vi "Main.vi"() -> ()   [LabVIEW 2013]
uses:
  ApplicationInititialisationClass/ApplicationInititialisation.lvclass
panel:
  out "error out":errorcluster
  out "Ergebnis-String":string
  out "VI-Name":string
  out "VI-Pfad":path
  out "WhereIGetMyInformation":string
  out "WhoIAm":string
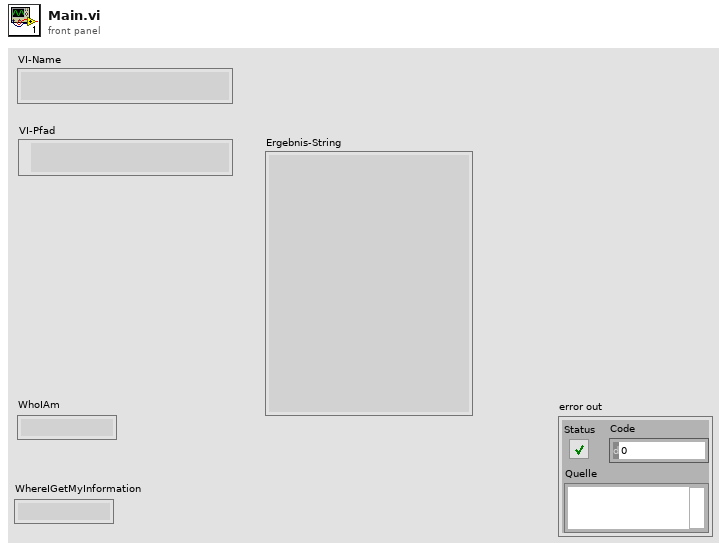
[diagram p1: front panel]
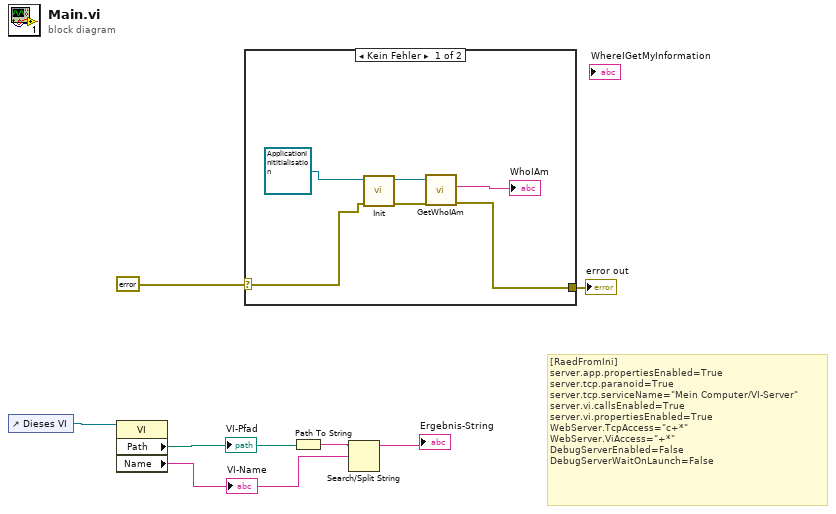
[diagram p0: block diagram]
diagram:
  # "[RaedFromIni]\nserver.app.propertiesEnabled=True\nserver.tcp.paranoid=True\nserver.tcp.serviceName=\"Mein Computer/VI-Server\"\nserver.vi.callsEnabled=True\nserver.vi.propertiesEnabled=True\nWebServer.TcpAccess=\"c+*\"\nWebServer.ViAccess=\"+*\"\nDebugServerEnabled=False\nDebugServerWaitOnLaunch=False"
  n1 = control-ref of="Dieses VI"() -> (w7:refnum<vi>)
  n2 = property class="VI"(reference=w7) -> ("Path"=w6:path, "Name"=w4:string)  [unwired: 1 in, 2 out]
  "VI-Pfad" <- w6
  "VI-Name" <- w4
  n3 = case shown="Kein Fehler" errorcluster {"status"=FALSE, "code"=0, "source"=""} ("error in (no error)") {
    selector: errorcluster {"status"=FALSE, "code"=0, "source"=""} ("error in (no error)") -> [w8 w14]
    tunnel: [w12 w14] -> w1
    frame No Error {
      n4 = call-dynamic "Init.vi"("error in (no error)"=w8, "ApplicationInititialisation Eingang"=refnum<class "ApplicationInititialisation.lvclass"> refnum ("ApplicationInititialisation.lvclass")) -> ("error out"=w9:errorcluster, "ApplicationInititialisation Ausgang"=w10:refnum<class "ApplicationInititialisation.lvclass">)  [unwired: 8 in]
      n5 = call-dynamic "GetWhoIAm .vi"("error in (no error)"=w9, "ApplicationInititialisation (Eingang)"=w10) -> ("error out"=w12:errorcluster, "WhoIAmData"=→"WhoIAm":string)  [unwired: 7 in, 1 out]
    }
    frame Error {
    }
  }
  "error out" <- w1
  n6 = Path To String(path=w6) -> (string=w5:string)
  n7 = Search/Split String(string=w5, search string/char (-)=w4) -> (substring before match=→"Ergebnis-String":string)  [unwired: 1 in, 2 out]
